vi "SetGenNOscL1.vi"(5 "Input Voltage":dbl=1.0, 7 "Enable Output":bool=TRUE, 8 "error in (no error)":errorcluster, 10 "VISA resource name":refnum<visa-resource-name>="AgilentOsciloscope", 11 "AWG VISA":refnum<visa-resource-name>="AgilentGenerator1") -> (0 "error out 2":errorcluster)   [LabVIEW 2012]
uses:
  Sum_Abrilader/L0_Sum_Adder Folder/C/Program Files/National Instruments/LabVIEW 2012/instr.lib/Agilent 81150/Agilent 81150.lvlib
  <instrlib>/Agilent 8000 Series/Agilent 8000 Series.lvlib
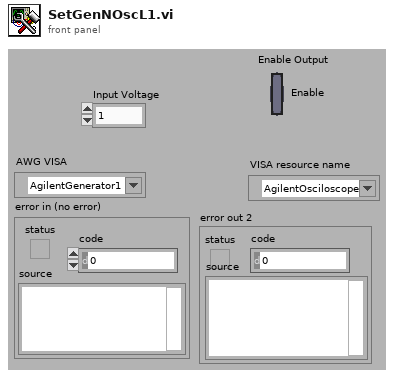
[diagram p1: front panel]
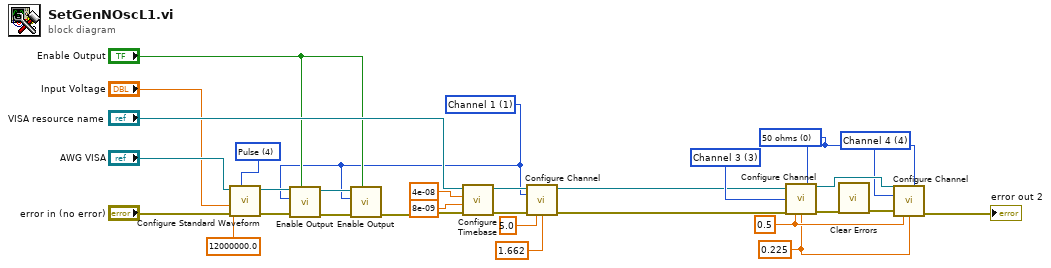
[diagram p0: block diagram]
diagram:
  w8 = 0.225 ("Vertical Offset (0.0 V)")
  w9 = 0.5 ("Vertical Range (2.0 V)")
  w19 = u32 0 items=["50 ohms", "1 Mohms"] ("Input Impedance (1: 1 Mohms)")
  w17 = 3 items=["Channel 1"=1, "Channel 2"=2, "Channel 3"=3, "Channel 4"=4] ("Channel (1: Channel 1)")
  w16 = 4 items=["Channel 1"=1, "Channel 2"=2, "Channel 3"=3, "Channel 4"=4] ("Channel (1: Channel 1)")
  w1 = 1 items=["Channel 1"=1, "Channel 2"=2, "Channel 3"=3, "Channel 4"=4] ("Channel (1: Channel 1)")
  w30 = u16 4 items=["Sine", "Square", "Ramp Up", "Ramp Down", "Pulse", "Noise", "DC"] ("Waveform (0: Sine)")
  n1 = call <instrlib>:"Configure Standard Waveform.vi"("Frequency (1000.0 Hz)"=12000000.0, "Waveform (0: Sine)"=w30, "error in (no error)"="error in (no error)", "Amplitude (1.0 Vpp)"="Input Voltage", "VISA resource name"="AWG VISA") -> ("error out"=w7:errorcluster, "VISA resource name out"=w6:refnum<visa-resource-name>)  [unwired: 5 in]
  n2 = call <instrlib>:"Enable Output.vi"("Enable Output (T: Enable)"="Enable Output", "error in (no error)"=w7, "Channel (1: Channel1)"=w1, "VISA resource name"=w6) -> ("error out"=w5:errorcluster, "VISA resource name out"=w3:refnum<visa-resource-name>)  [unwired: 6 in]
  n3 = call <instrlib>:"Enable Output.vi"("Enable Output (T: Enable)"="Enable Output", "error in (no error)"=w5, "Channel (1: Channel1)"=w1, "VISA resource name"=w3) -> ("error out"=w4:errorcluster)  [unwired: 6 in, 1 out]
  n4 = call "Configure Timebase.vi"("error in (no error)"=w4, "Position (0.0 s)"=8e-09, "Timebase (0.005 s)"=4e-08, "VISA resource name"="VISA resource name") -> ("error out"=w28:errorcluster, "VISA resource name out"=w27:refnum<visa-resource-name>)  [unwired: 6 in]
  n5 = call <instrlib>:"Configure Channel.vi"("VISA resource name"=w27, "Channel (1: Channel 1)"=w1, "error in (no error)"=w28, "Vertical Range (2.0 V)"=5.0, "Vertical Offset (0.0 V)"=1.662) -> ("VISA resource name out"=w15:refnum<visa-resource-name>, "error out"=w14:errorcluster)  [unwired: 9 in]
  n6 = call <instrlib>:"Configure Channel.vi"("VISA resource name"=w15, "Input Impedance (1: 1 Mohms)"=w19, "Channel (1: Channel 1)"=w17, "error in (no error)"=w14, "Vertical Range (2.0 V)"=w9, "Vertical Offset (0.0 V)"=w8) -> ("VISA resource name out"=w20:refnum<visa-resource-name>, "error out"=w21:errorcluster)  [unwired: 8 in]
  n7 = call <vilib>:"Clear Errors.vi"("error in (no error)"=w21) -> ("error out"=w18:errorcluster)  [unwired: 6 in]
  n8 = call <instrlib>:"Configure Channel.vi"("VISA resource name"=w20, "Input Impedance (1: 1 Mohms)"=w19, "Channel (1: Channel 1)"=w16, "error in (no error)"=w18, "Vertical Range (2.0 V)"=w9, "Vertical Offset (0.0 V)"=w8) -> ("error out"=→"error out 2":errorcluster)  [unwired: 8 in, 1 out]
